vi "SetDeltaT.vi"(8 "error in (no error)":errorcluster) -> (0 "error out":errorcluster)   [LabVIEW 2019, in "RT_Game.lvlib" / "Engine.lvclass"]
uses:
  Engine.lvclass
  Globals.vi
  RT_Game.lvlib
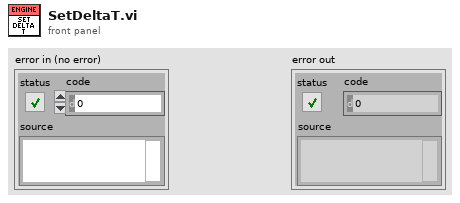
[diagram p1: front panel]
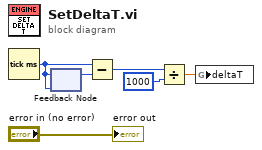
[diagram p0: block diagram]
diagram:
  n1 = Tick Count (ms)() -> (millisecond timer value=w3:u32)
  n2 = feedback #1(w3) -> (w2:u32)
  n3 = feedback-in #1(w3) -> ()
  n4 = Subtract(x=w3, y=w2) -> (x-y=w4:u32)
  n5 = Divide(x=w4, y=u32 1000) -> (x/y=w6:dbl)
  n6 = global write "Globals.vi" "deltaT"(w6) -> ()
  "error out" <- "error in (no error)"
